vi "MT_DATA Pro (SubVI).vi"(4 "mag_n":dbl[](array[numeric])=[0.25, 0.0, 0.85], 5 "Initialize":bool, 6 "h":dbl=0.2, 7 "K_i":dbl[][](array[numeric])=[[0.05, 0.0, 0.0], [0.0, 0.05, 0.0], [0.0, 0.0, 0.05]], 8 "K_p":dbl[][](array[numeric])=[[2.0, 0.0, 0.0], [0.0, 2.0, 0.0], [0.0, 0.0, 40.0]], 9 "k_mes":dbl[](array[numeric])=[1.0, 1.0], 10 "MT_SINGLE":sgl[](array[numeric])=[-0.117490456, -0.46173555, -9.88218, 0.005892315, -0.0058561633, 0.0012556299, 0.075646125, -0.7224537, -0.16176447, 2.5945768, -0.61170423, 84.21202]) -> (0 "THETA_hat":dbl[](array[numeric]), 1 "bg":dbl[](array[numeric]), 2 "omega_hat":dbl[](array[numeric]), 3 "THETA_mes":dbl[](array[numeric]))   [LabVIEW 2014, in "Observer Library.lvlib" / "Attitude Observer.lvclass"]
uses:
  Attitude Observer.lvclass
  <vilib>/imath/engines/lvmath2/RunTimeEngine/IndexRead/NIMS V(S).vi
  <instcachedir>/0/NIMS V(S)_0488751826AF41519A22953C041130DC.lvgen/NIMS V(S)_0488751826AF41519A22953C041130DC_004.vi
  <vilib>/imathl/engines/lvmath/Functions/Error Handling/Create Error.vi
  <vilib>/imath/engines/lvmath2/RunTimeEngine/BuiltInFunctions/atan2/NIMS_atan2.vi
  <instcachedir>/0/NIMS_atan2_A91AA4A7D42247EDBE8F76DB99AF04A4.lvgen/NIMS_atan2_A91AA4A7D42247EDBE8F76DB99AF04A4_002.vi
  <vilib>/imath/engines/lvmath2/RunTimeEngine/BuiltInFunctions/abs/NIMS_abs(signed).vi
  <instcachedir>/0/NIMS_abs(signed)_C4FCB8E6058B49B797C7C8D53CA5F6EC.lvgen/NIMS_abs(signed)_C4FCB8E6058B49B797C7C8D53CA5F6EC_000.vi
  <instcachedir>/0/NIMS_atan2_A91AA4A7D42247EDBE8F76DB99AF04A4.lvgen/NIMS_atan2_A91AA4A7D42247EDBE8F76DB99AF04A4_003.vi
  <vilib>/imath/engines/lvmath2/RunTimeEngine/ArithmeticOperatorToken/NIMS_ArithmeticOperator_multmx-internal.vi
  <instcachedir>/0/NIMS_ArithmeticOperator_multmx-internal_D7C5C88E94B94895A818D3A8E50A4506.lvgen/NIMS_ArithmeticOperator_multmx-internal_D7C5C88E94B94895A818D3A8E50A4506_014.vi
  <vilib>/imath/engines/lvmath2/RunTimeEngine/ArithmeticOperatorToken/NIMS_ArithmeticOperator_multmx(M,CV)-internal.vi
  <instcachedir>/0/NIMS_ArithmeticOperator_multmx(M,CV)-internal_25C7CE5937BA4322B5BE2717374345EA.lvgen/NIMS_ArithmeticOperator_multmx(M,CV)-internal_25C7CE5937BA4322B5BE2717374345EA_002.vi
  <vilib>/imath/engines/lvmath2/RunTimeEngine/ErrorHandling/NIMS_Create Error From Enums.vi
  <instcachedir>/0/NIMS V(S)_0488751826AF41519A22953C041130DC.lvgen/NIMS V(S)_0488751826AF41519A22953C041130DC_000.vi
  <instcachedir>/0/NIMS_atan2_A91AA4A7D42247EDBE8F76DB99AF04A4.lvgen/NIMS_atan2_A91AA4A7D42247EDBE8F76DB99AF04A4_000.vi
  <instcachedir>/0/NIMS_ArithmeticOperator_multmx-internal_D7C5C88E94B94895A818D3A8E50A4506.lvgen/NIMS_ArithmeticOperator_multmx-internal_D7C5C88E94B94895A818D3A8E50A4506_015.vi
  <instcachedir>/0/NIMS_ArithmeticOperator_multmx-internal_D7C5C88E94B94895A818D3A8E50A4506.lvgen/NIMS_ArithmeticOperator_multmx-internal_D7C5C88E94B94895A818D3A8E50A4506_004.vi
  <vilib>/imath/engines/lvmath2/RunTimeEngine/IndexRead/NIMS V(R2).vi
  <instcachedir>/0/NIMS V(R2)_C76619605A0E4E9F8B2FA9389712AC47.lvgen/NIMS V(R2)_C76619605A0E4E9F8B2FA9389712AC47_000.vi
  <vilib>/imath/engines/lvmath2/RunTimeEngine/ArithmeticOperatorToken/NIMS_ArithmeticOperator_powermx(M,M).vi
  <vilib>/imath/engines/lvmath/Functions/Error Handling/MergeErrorsWrapper.vi
  <instcachedir>/0/NIMS_ArithmeticOperator_multmx(M,CV)-internal_25C7CE5937BA4322B5BE2717374345EA.lvgen/NIMS_ArithmeticOperator_multmx(M,CV)-internal_25C7CE5937BA4322B5BE2717374345EA_007.vi
  <instcachedir>/0/NIMS_ArithmeticOperator_multmx(M,CV)-internal_25C7CE5937BA4322B5BE2717374345EA.lvgen/NIMS_ArithmeticOperator_multmx(M,CV)-internal_25C7CE5937BA4322B5BE2717374345EA_008.vi
  <instcachedir>/0/NIMS_ArithmeticOperator_multmx-internal_D7C5C88E94B94895A818D3A8E50A4506.lvgen/NIMS_ArithmeticOperator_multmx-internal_D7C5C88E94B94895A818D3A8E50A4506_012.vi
  <instcachedir>/0/NIMS_ArithmeticOperator_multmx-internal_D7C5C88E94B94895A818D3A8E50A4506.lvgen/NIMS_ArithmeticOperator_multmx-internal_D7C5C88E94B94895A818D3A8E50A4506_016.vi
  <vilib>/imath/engines/lvmath2/RunTimeEngine/IndexRead/NIMS M(S,S).vi
  <instcachedir>/0/NIMS M(S,S)_AC51E74150A542F7991B9634C66F3096.lvgen/NIMS M(S,S)_AC51E74150A542F7991B9634C66F3096_001.vi
  <instcachedir>/0/NIMS M(S,S)_AC51E74150A542F7991B9634C66F3096.lvgen/NIMS M(S,S)_AC51E74150A542F7991B9634C66F3096_000.vi
  <vilib>/imath/engines/lvmath2/RunTimeEngine/ArithmeticOperatorToken/NIMS_ArithmeticOperator_multmx(M,CV).vi
  <instcachedir>/0/NIMS_ArithmeticOperator_multmx(M,CV)_787B4652E60B4C52835A7FB23671E425.lvgen/NIMS_ArithmeticOperator_multmx(M,CV)_787B4652E60B4C52835A7FB23671E425_005.vi
  <vilib>/imath/engines/lvmath2/RunTimeEngine/ArithmeticOperatorToken/NIMS_ArithmeticOperator_minus.vi
  <instcachedir>/0/NIMS_ArithmeticOperator_minus_39C0593E74DA4138ACA2AB742906488D.lvgen/NIMS_ArithmeticOperator_minus_39C0593E74DA4138ACA2AB742906488D_010.vi
  <instcachedir>/0/NIMS_ArithmeticOperator_minus_39C0593E74DA4138ACA2AB742906488D.lvgen/NIMS_ArithmeticOperator_minus_39C0593E74DA4138ACA2AB742906488D_011.vi
  <vilib>/imath/engines/lvmath2/RunTimeEngine/ArithmeticOperatorToken/NIMS_ArithmeticOperator_plus.vi
  <instcachedir>/0/NIMS_ArithmeticOperator_plus_48D6EAACA5D645B09F7EC9C016C2DEA8.lvgen/NIMS_ArithmeticOperator_plus_48D6EAACA5D645B09F7EC9C016C2DEA8_002.vi
  <vilib>/imath/engines/lvmath2/RunTimeEngine/ArithmeticOperatorToken/NIMS_ArithmeticOperator_multmx.vi
  <instcachedir>/0/NIMS_ArithmeticOperator_multmx_CE3986B82B8C4E94A31593A7EF82383B.lvgen/NIMS_ArithmeticOperator_multmx_CE3986B82B8C4E94A31593A7EF82383B_009.vi
  <instcachedir>/0/NIMS_ArithmeticOperator_plus_48D6EAACA5D645B09F7EC9C016C2DEA8.lvgen/NIMS_ArithmeticOperator_plus_48D6EAACA5D645B09F7EC9C016C2DEA8_010.vi
  <instcachedir>/0/NIMS_ArithmeticOperator_multmx_CE3986B82B8C4E94A31593A7EF82383B.lvgen/NIMS_ArithmeticOperator_multmx_CE3986B82B8C4E94A31593A7EF82383B_003.vi
  <vilib>/imath/engines/lvmath2/RunTimeEngine/ArithmeticOperatorToken/NIMS_ArithmeticOperator_rightdivmx(C,C).vi
  <instcachedir>/0/NIMS_ArithmeticOperator_rightdivmx(C,C)_AEA1716F6A4941D8B61B119A3B266D0E.lvgen/NIMS_ArithmeticOperator_rightdivmx(C,C)_AEA1716F6A4941D8B61B119A3B266D0E_000.vi
  <vilib>/imath/engines/lvmath2/RunTimeEngine/IndexRead/NIMS M(S).vi
  <instcachedir>/0/NIMS M(S)_B826C018497E4940AE96BD27B540B6FB.lvgen/NIMS M(S)_B826C018497E4940AE96BD27B540B6FB_004.vi
  <vilib>/imath/engines/lvmath2/RunTimeEngine/IndexRead/NIMS M(R2).vi
  <instcachedir>/0/NIMS M(R2)_287818D58BD74005B29FE73CE7602B1A.lvgen/NIMS M(R2)_287818D58BD74005B29FE73CE7602B1A_001.vi
  <instcachedir>/0/NIMS_atan2_A91AA4A7D42247EDBE8F76DB99AF04A4.lvgen/NIMS_atan2_A91AA4A7D42247EDBE8F76DB99AF04A4_001.vi
  <vilib>/imath/engines/lvmath2/RunTimeEngine/BuiltInFunctions/asin/NIMS_asin(C).vi
  <instcachedir>/0/NIMS_asin(C)_7FBCC14D953545E18098594EA458D330.lvgen/NIMS_asin(C)_7FBCC14D953545E18098594EA458D330_001.vi
  <vilib>/imath/engines/lvmath2/RunTimeEngine/NodeEndStatement/NIMS_NodeEndStatement_Get Vector.vi
  <instcachedir>/0/NIMS_NodeEndStatement_Get Vector_00D1625602D843AD9D7EC134A9EC13A2.lvgen/NIMS_NodeEndStatement_Get Vector_00D1625602D843AD9D7EC134A9EC13A2_003.vi
  <vilib>/imath/engines/lvmath2/RunTimeEngine/NodeEndStatement/NIMS_NodeEndStatement_Output.vi
  <instcachedir>/0/NIMS_NodeEndStatement_Output_53EC0D466D134D7ABD903AC30B43404B.lvgen/NIMS_NodeEndStatement_Output_53EC0D466D134D7ABD903AC30B43404B_005.vi
  <instcachedir>/0/NIMS_NodeEndStatement_Output_53EC0D466D134D7ABD903AC30B43404B.lvgen/NIMS_NodeEndStatement_Output_53EC0D466D134D7ABD903AC30B43404B_001.vi
  <instcachedir>/0/NIMS_NodeEndStatement_Output_53EC0D466D134D7ABD903AC30B43404B.lvgen/NIMS_NodeEndStatement_Output_53EC0D466D134D7ABD903AC30B43404B_000.vi
  <instcachedir>/0/NIMS_NodeEndStatement_Output_53EC0D466D134D7ABD903AC30B43404B.lvgen/NIMS_NodeEndStatement_Output_53EC0D466D134D7ABD903AC30B43404B_017.vi
  <instcachedir>/0/NIMS_NodeEndStatement_Output_53EC0D466D134D7ABD903AC30B43404B.lvgen/NIMS_NodeEndStatement_Output_53EC0D466D134D7ABD903AC30B43404B_003.vi
  <vilib>/imath/engines/lvmath2/RunTimeEngine/ErrorHandling/NIMS_Finalize Error.vi
panel:
  in  "T_f":dbl=15.0
  in  "k_is":dbl=1.0
  out "v_2b_hat":dbl[](array[numeric])
  out "v_2b":dbl[](array[numeric])
  out "v_1b_hat":dbl[](array[numeric])
  out "v_1b":dbl[](array[numeric])
  out "omega_mes":dbl[](array[numeric])
  out "temp":dbl[][](array[numeric])
  out "q_hat":dbl[](array[numeric])
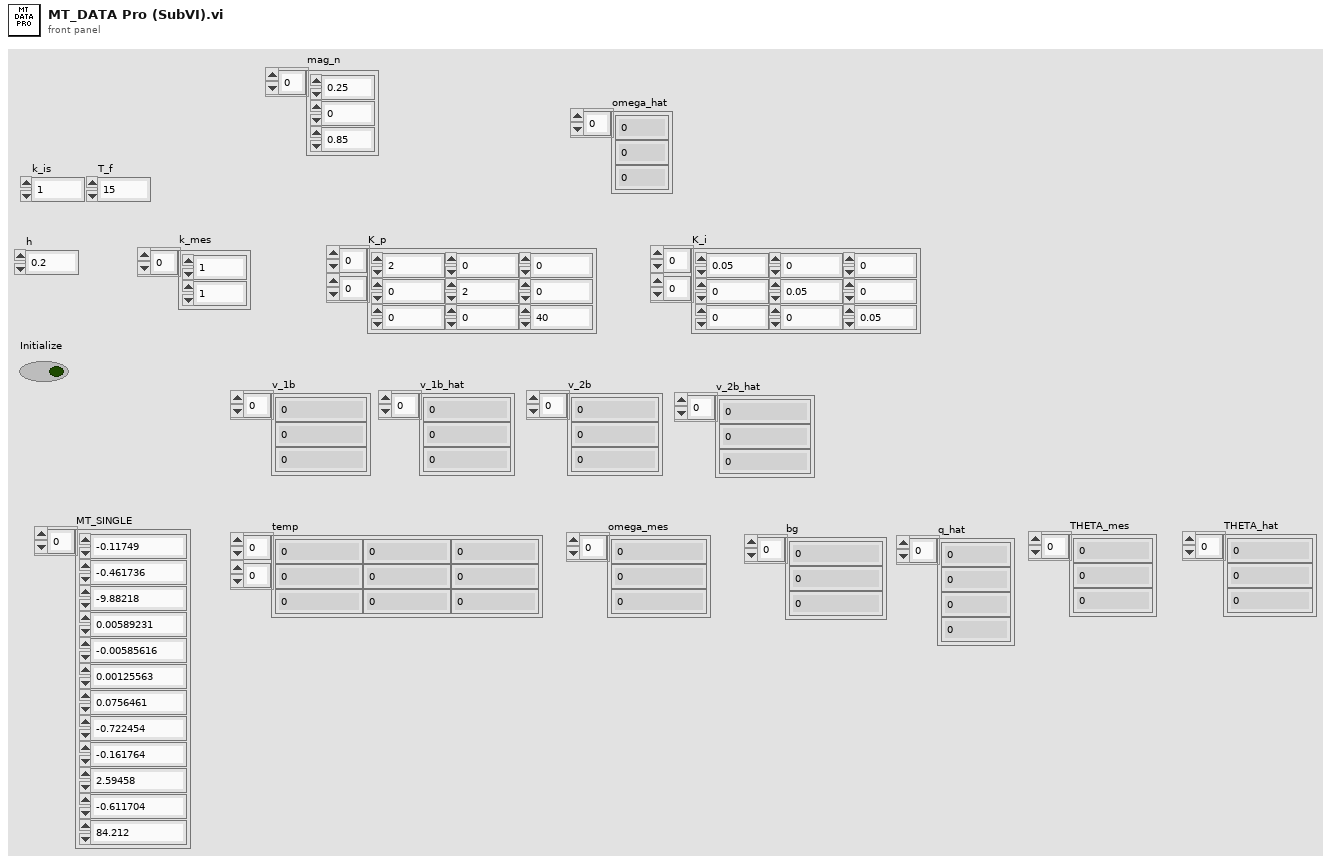
[diagram p1: front panel]
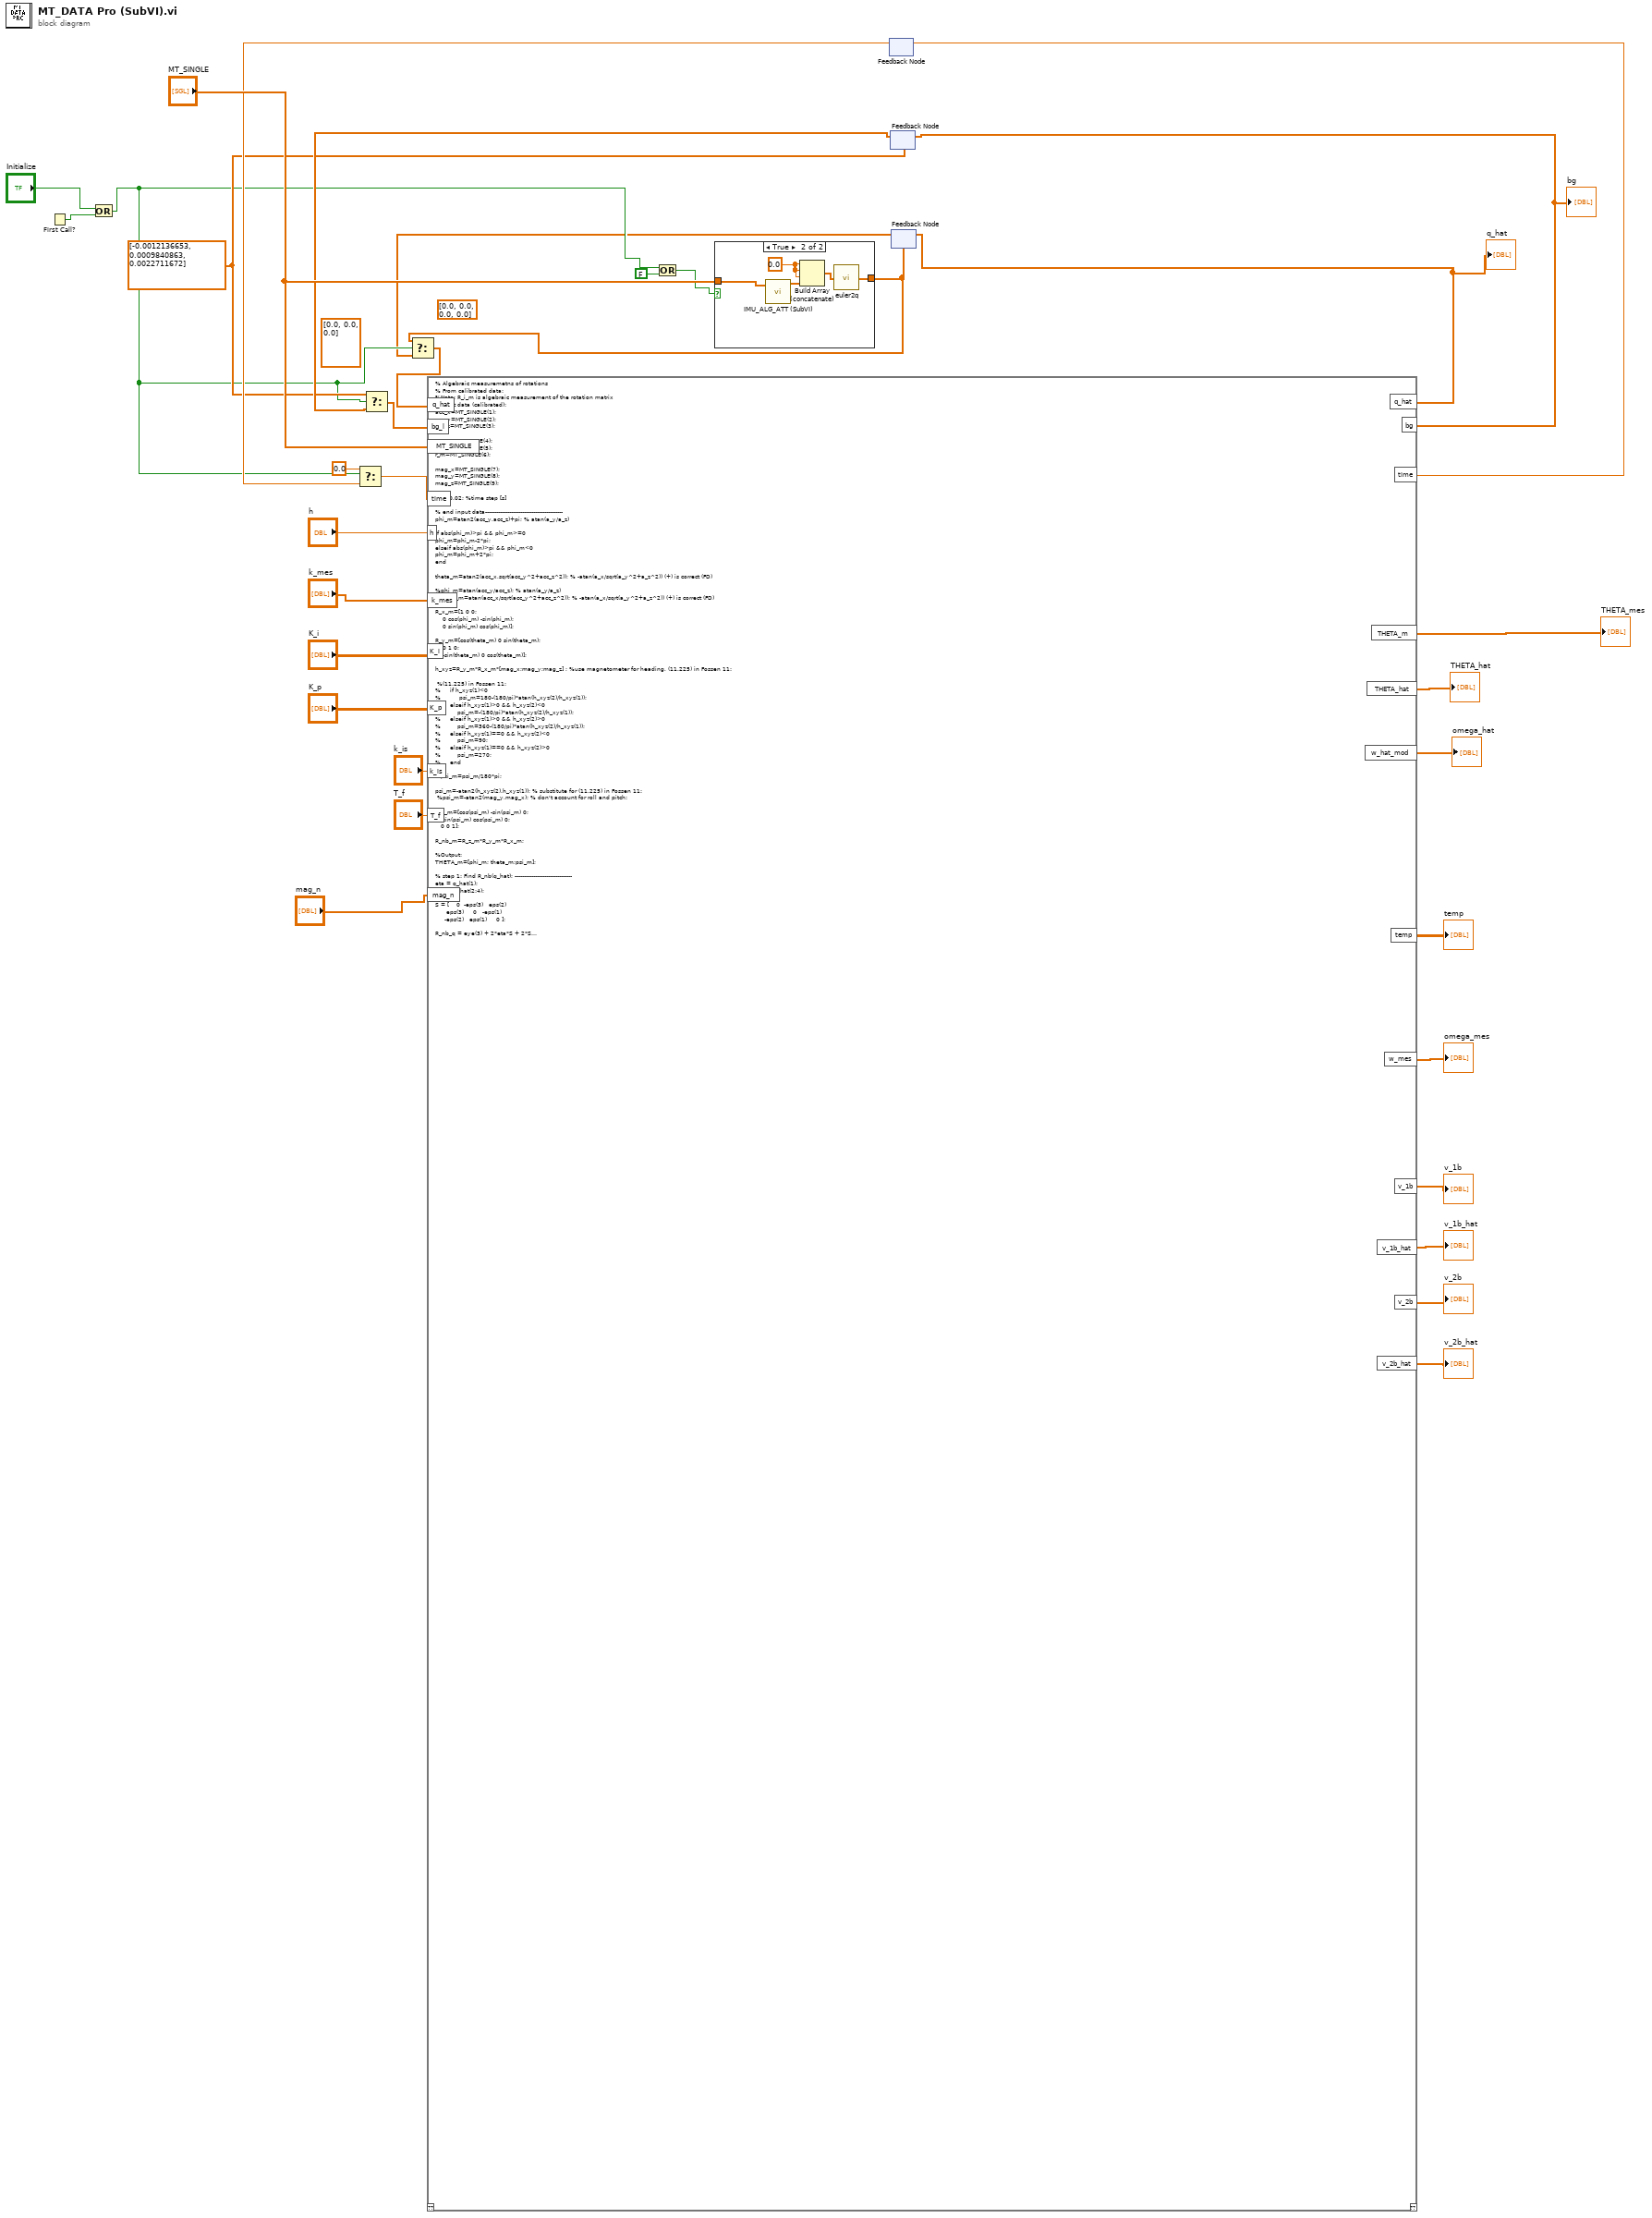
[diagram p0: block diagram]
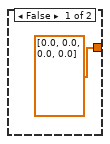
[diagram p2: hidden frame]
diagram:
  (unwired) dbl[] [0.0, 0.0, 0.0, 0.0]
  (unwired) dbl[] [0.0, 0.0, 0.0] ("bg")
  w11 = dbl[] [-0.0012136653, 0.0009840863, 0.0022711672] ("bg")
  n1 = First Call?() -> (First Call?: T/F=w6:bool)
  n2 = Or(x="Initialize", y=w6) -> (x .or. y?=w3:bool)
  n3 = Or(x=w3, y=FALSE) -> (x .or. y?=w8:bool)
  n4 = case shown="True" w8 {
    tunnel: "MT_SINGLE" -> [_ w40]
    tunnel: [dbl[] [0.0, 0.0, 0.0, 0.0] ("q") w39] -> w1
    frame False {
    }
    frame True {
      w37 = 0.0
      n5 = call "IMU_ALG_ATT (SubVI).vi"("MT_SINGLE"=w40) -> ("THETA_m"=w38:dbl[])  [unwired: 10 in]
      n6 = Build Array (concatenate)(w37, w37, w37, w38) -> (w36:dbl[])
      n7 = call "euler2q.vi"("Eta"=w36) -> ("q"=w39:dbl[])
    }
  }
  n8 = feedback #1() -> (w18:dbl)  [unwired: 1 in]
  n9 = Select(t=0.0, s=w3, f=w18) -> (s? t:f=w16:dbl)
  n10 = feedback #2(w11) -> (w14:dbl[])
  n11 = Select(t=w11, s=w3, f=w14) -> (s? t:f=w15:dbl[])
  n12 = feedback #3(w1) -> (w2:dbl[])
  n13 = Select(t=w1, s=w3, f=w2) -> (s? t:f=w4:dbl[])
  n14 = mathscript code="% Algebraic measuremetns of rotations\n% From calibrated data:\n%Note: R_i_m is algebraic measurement of the rotation matrix\n%input data (calibrated):\nacc_x=MT_SINGLE(1);\nacc_y=MT_SINGLE(2);\nacc_z=MT_SINGLE(3);\n\np_m=MT_SINGLE(4);\nq_m=MT_SINGLE(5);\nr_m=MT_SINGLE(6);\n\nmag_x=MT_SINGLE(7);\nmag_y=MT_SINGLE(8);\nmag_z=MT_SINGLE(9);\n\n%h=0.02; %time step [s] \n\n% end input data------------------------------------------\nphi_m=atan2(acc_y,acc_z)+pi; % atan(a_y/a_z)\n\nif abs(phi_m)>pi && phi_m>=0\nphi_m=phi_m-2*pi;\nelseif abs(phi_m)>pi && phi_m<0\nphi_m=phi_m+2*pi;  \nend\n\ntheta_m=atan2(acc_x,sqrt(acc_y^2+acc_z^2)); % -atan(a_x/sqrt(a_y^2+a_z^2)) (+) is correct (FD) \n\n%phi_m=atan(acc_y/acc_z); % atan(a_y/a_z)\n%theta_m=atan(acc_x/sqrt(acc_y^2+acc_z^2)); % -atan(a_x/sqrt(a_y^2+a_z^2)) (+) is correct (FD) \n    \nR_x_m=[1 0 0;\n    0 cos(phi_m) -sin(phi_m);\n    0 sin(phi_m) cos(phi_m)];    \n    \nR_y_m=[cos(theta_m) 0 sin(theta_m);\n    0 1 0;\n    -sin(theta_m) 0 cos(theta_m)];\n\nh_xyz=R_y_m*R_x_m*[mag_x;mag_y;mag_z] ; %use magnetometer for heading, (11.225) in Fossen 11:\n\n %(11.225) in Fossen 11:\n%     if h_xyz(1)<0\n%          psi_m=180-(180/pi)*atan(h_xyz(2)/h_xyz(1));\n%     elseif h_xyz(1)>0 && h_xyz(2)<0\n%         psi_m=-(180/pi)*atan(h_xyz(2)/h_xyz(1));\n%     elseif h_xyz(1)>0 && h_xyz(2)>0\n%         psi_m=360-(180/pi)*atan(h_xyz(2)/h_xyz(1));\n%     elseif h_xyz(1)==0 && h_xyz(2)<0\n%         psi_m=90;\n%     elseif h_xyz(1)==0 && h_xyz(2)>0\n%         psi_m=270;\n%     end\n\n%psi_m=psi_m/180*pi;\n\npsi_m=-atan2(h_xyz(2),h_xyz(1)); % substitute for (11.225) in Fossen 11:\n %psi_m=-atan2(mag_y,mag_x); % don't account for roll and pitch:\n\nR_z_m=[cos(psi_m) -sin(psi_m) 0;\n    sin(psi_m) cos(psi_m) 0;\n   0 0 1];    \n\nR_nb_m=R_z_m*R_y_m*R_x_m;  \n\n%Output:\nTHETA_m=[phi_m; theta_m;psi_m]; \n\n% step 1: Find R_nb(q_hat); -------------------------------\neta = q_hat(1);\neps = q_hat(2:4);\n\nS = [    0  -eps(3)   eps(2)\n      eps(3)     0   -eps(1)\n     -eps(2)   eps(1)     0 ];\n\nR_nb_q = eye(3) + 2*eta*S + 2*S^2;\n% end step 1--------------------------------------------------\n\n% step 2: Find normalized acceleration and magnetometer measurements ; -----------------\nv_1b=[acc_x;acc_y;acc_z]/sqrt(acc_x^2+acc_y^2+acc_z^2);  % (11.299)\nv_2b=[mag_x;mag_y;mag_z]/sqrt(mag_x^2+mag_y^2+mag_z^2); % (11.299)\n% end step 2--------------------------------------------------\n\n% step 3: Find estimate of v_ib:\nv_1b_hat=R_nb_q'*[0;0;-1] ;  % (11.306) in Fossen 11 (Note change in sign to -1 and transpose.)\n\n%mag_nx=0.26;\n%mag_ny=0;\n%mag_nz=0.84;\nmag_nx=mag_n(1);\nmag_ny=mag_n(2);\nmag_nz=mag_n(3);\n\nv_2b_hat=R_nb_q'*[mag_nx;mag_ny;mag_nz]/sqrt(mag_nx^2+mag_ny^2+mag_nz^2); % (11.308) in Fossen 11 (Note change to ned and transpose)\n% end step 3------------------------------------------------------------------------\n\n%step 4: find w_mes_b :--------------------------------------------------\ntemp=0.5*k_mes(1)*(v_1b*v_1b_hat'-v_1b_hat*v_1b')+0.5*k_mes(2)*(v_2b*v_2b_hat'-v_2b_hat*v_2b');\nw_mes=-[temp(3,2);temp(1,3);temp(2,1)];\n%end step 4------------------------------------------------------------------------\n\n%step 5: find bias gyro :--------------------------------------------------\nif time<100\nK_it=K_i*(1+(k_is/K_i(1,1)-1))*exp(-(time)/T_f);\nelse\nK_it=K_i;\nend\n\ntime=time+h;\n\nbg=bg_l'-h*0.5*K_it*w_mes;   %NOTE: transpose because of labview convetion (bg=bg_l'-h*0.5*K_i*w_mes; )\n%end step 5------------------------------------------------------------------------\n\n%step 6: find T(q) :--------------------------------------------------\n%eta  = q(1); eps1 = q(2); eps2 = q(3); eps3 = q(4); \nT_q = 0.5*[...\n   -eps(1) -eps(2) -eps(3)        \n    eta  -eps(3)  eps(2)\n    eps(3)  eta  -eps(1)\n   -eps(2)  eps(1)  eta ];\n%end step 6------------------------------------------------------------------------\n\n%step 7: find q:--------------------------------------------------\nw_imu=[p_m;q_m;r_m]; %[rads/s]\nw_hat=w_imu-bg+K_p*w_mes;\n\nq_hat=q_hat'+h*T_q*w_hat;   %NOTE: transpose because of labview convetion\n\nq_hat=q_hat/sqrt(q_hat'*q_hat); \n%end step 7------------------------------------------------------------------------\n\n%step 7: quaternions to euler angles::--------------------------------------------------\n\neta = q_hat(1);\neps = q_hat(2:4);\n\nS = [ 0  -eps(3)   eps(2)\n      eps(3)     0   -eps(1)\n     -eps(2)   eps(1)     0 ];\n\nR= eye(3) + 2*eta*S + 2*S^2;\n \nphi_h   = atan2(R(3,2),R(3,3));\ntheta_h = -asin(R(3,1));\npsi_h   = atan2(R(2,1),R(1,1));\n\nTHETA_hat=[phi_h;theta_h;psi_h]; \n\nw_hat_mod=w_imu-bg;"("MT_SINGLE"="MT_SINGLE", "q_hat"=w4, "bg_l"=w15, "h"="h", "k_mes"="k_mes", "K_i"="K_i", "K_p"="K_p", "time"=w16, "k_is"="k_is", "T_f"="T_f", "mag_n"="mag_n") -> ("THETA_m"=→"THETA_mes":dbl[], "q_hat"=w30:dbl[], "temp"=→"temp":cdb[][], "w_mes"=→"omega_mes":cdb[], "bg"=w29:dbl[], "THETA_hat"=→"THETA_hat":cdb[], "v_1b"=→"v_1b":csg[], "v_1b_hat"=→"v_1b_hat":cdb[], "v_2b"=→"v_2b":csg[], "v_2b_hat"=→"v_2b_hat":cdb[], "time"=w19:dbl, "w_hat_mod"=→"omega_hat":dbl[])  [unwired: 1 in, 1 out]
  "q_hat" <- w30
  "bg" <- w29
  n15 = feedback-in #1(w19) -> ()
  n16 = feedback-in #2(w29) -> ()
  n17 = feedback-in #3(w30) -> ()
